vi "IVTcpLV2.vi"(4 "数值类型":enum16{"长整型", "双精度"}(ring), 6 "TCP连接参数":cluster{"IP地址":string, "端口":u16}={"IP地址"="10.232.43.160", "端口"=502}, 7 "TCP操作模式":enum16{"打开TCP", "读MW区", "写MW区", "关闭TCP"}(ring), 8 "错误输入":errorcluster, 9 "值":dbl format="%.3g", 10 "值":i32=10, 11 "寄存器MD地址":i32=10) -> (0 "错误输出":errorcluster, 1 "数值":sgl, 2 "数值":u32, 3 "=1？":bool)   [LabVIEW 2016]
panel:
  out "读写OK":bool
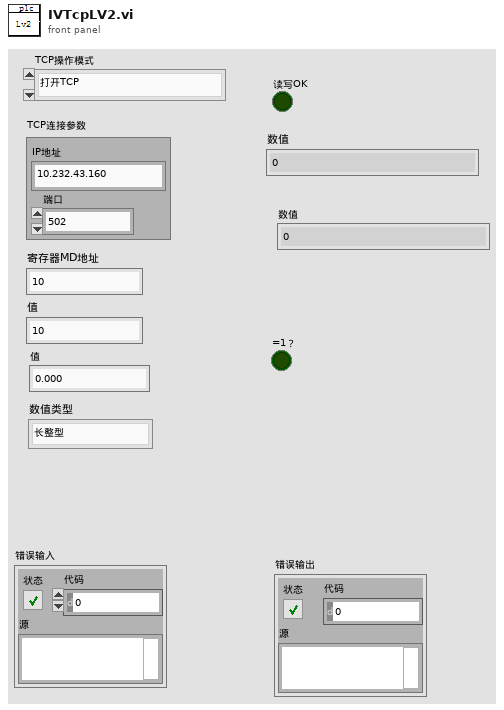
[diagram p1: front panel]
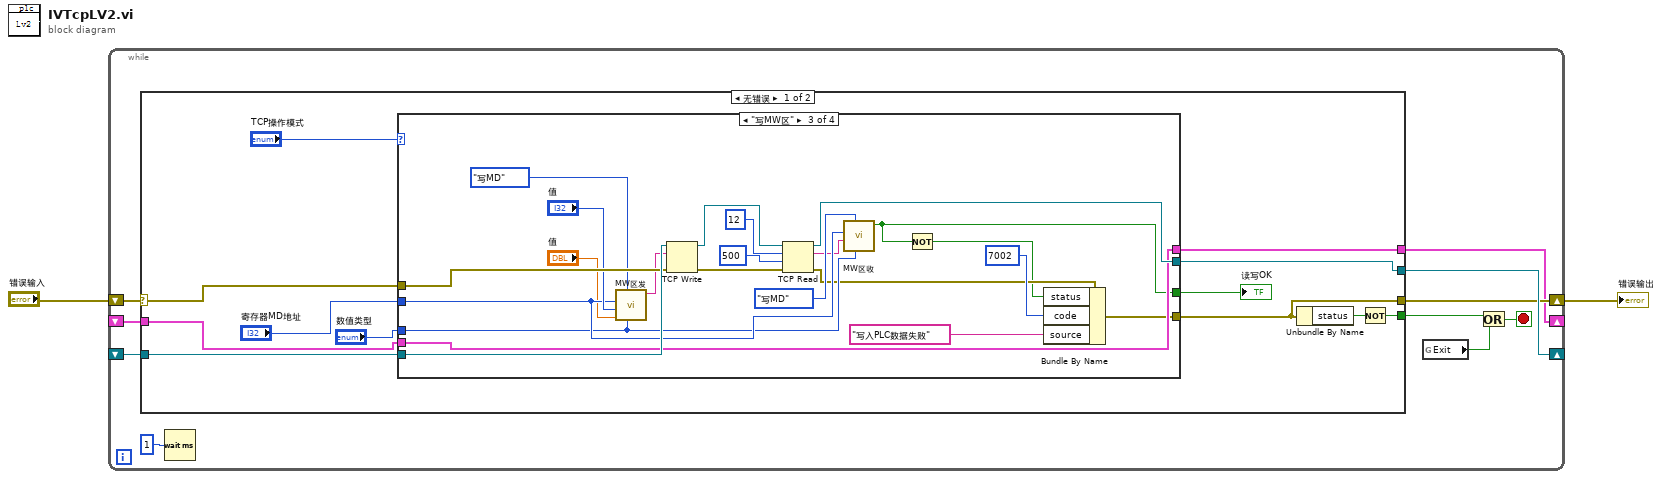
[diagram p0: block diagram]
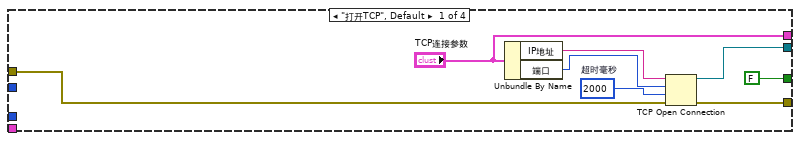
[diagram p2: hidden frame]
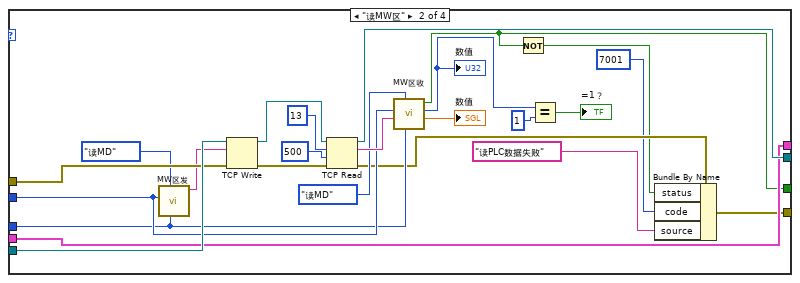
[diagram p3: hidden frame]
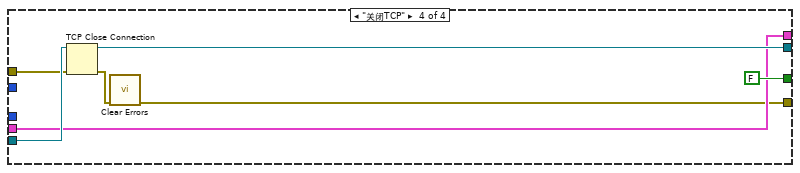
[diagram p4: hidden frame]
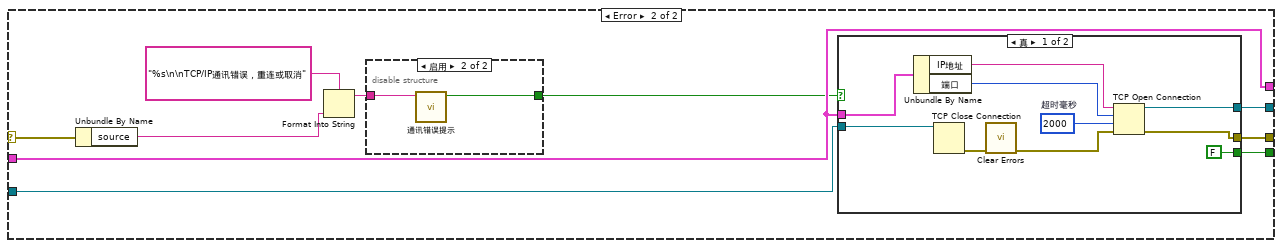
[diagram p5: hidden frame]
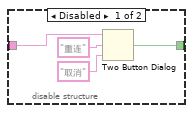
[diagram p6: hidden frame]
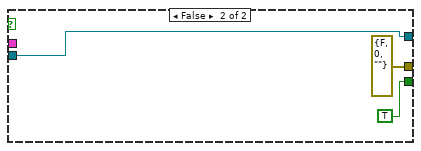
[diagram p7: hidden frame]
diagram:
  n1 = while {
    shift-right: [w6] -> w1
    shift-left: "错误输入" -> [w11]
    shift-right: [w10] -> _
    shift-left: _ -> [w12]
    shift-right: [w5] -> _
    shift-left: _ -> [w4]
    stop <- w8 stop-if-true
    n2 = case shown="无错误" w11 {
      selector: w11 -> [w18 w89]
      tunnel: w12 -> [w21 w94]
      tunnel: [w22 w95] -> w10
      tunnel: [w20 w93] -> w7
      tunnel: [w17 w92] -> w6
      tunnel: [w16 w91] -> w5
      tunnel: w4 -> [w15 w91]
      frame No Error {
        n3 = case shown="\"写MW区\"" "TCP操作模式" {
          tunnel: [FALSE ("读取OK") w36 w59 FALSE ("读取OK")] -> w24
          tunnel: [w31 w53 w74 w84] -> w22
          tunnel: w21 -> [_ w52 w75 w85]
          tunnel: [w30 w37 w57 w79] -> w17
          tunnel: w18 -> [w28 w51 w73 w81]
          tunnel: ["TCP连接参数" w50 w72 w82] -> w16
          tunnel: w15 -> [_ w50 w72 w82]
          tunnel: "寄存器MD地址" -> [_ w46 w67 _]
          tunnel: "数值类型" -> [_ w43 w63 _]
          frame "打开TCP", Default {
            w32 = 2000  # 超时毫秒
            n4 = Unbundle By Name("TCP连接参数") -> ("IP地址"=w27:string, "端口"=w26:u16)
            n5 = TCP Open Connection(address=w27, remote port or service name=w26, timeout ms (60000)=w32, error in (no error)=w28) -> (connection ID=w31:refnum<k5>, error out=w30:errorcluster)  [unwired: 1 in]
          }
          frame "读MW区" {
            n6 = call "MW区发.vi"("数值类型"=w43, "MD模式"=enum16{"读MD", "写MD"}."读MD", "寄存器MD地址"=w46) -> ("String"=w45:string)  [unwired: 8 in]
            n7 = TCP Write(connection ID=w52, data in=w45, error in (no error)=w51) -> (connection ID out=w56:refnum<k5>, error out=w55:errorcluster)  [unwired: 1 in, 1 out]
            n8 = TCP Read(connection ID=w56, bytes to read=13 ("读取的字节"), error in (no error)=w55, 9:500 ("超时毫秒(25000)")) -> (connection ID out=w53:refnum<k5>, data out=w48:string, error out=w38:errorcluster)  [unwired: 1 in]
            n9 = call "MW区收.vi"("数值类型"=w43, "MD模式"=enum16{"读MD", "写MD"}."读MD", "16#字符串"=w48, "寄存器MD地址"=w46) -> (1:"数值"=→"数值":sgl, 2:"数值"=w39:u32, "读写OK"=w36:bool)  [unwired: 5 in]
            "数值" <- w39
            n10 = Not(x=w36) -> (.not. x?=w35:bool)
            n11 = Equal?(x=w39, y=u32 1) -> (x = y?=→"=1？":bool)
            n12 = Bundle By Name(cluster=w38, "status"=w35, "code"=7001, "source"="读PLC数据失败") -> (w37:errorcluster)
          }
          frame "写MW区" {
            n13 = call "MW区发.vi"("数值类型"=w63, "MD模式"=enum16{"读MD", "写MD"}."写MD", 8:"值"="值", 9:"值"="值", "寄存器MD地址"=w67) -> ("String"=w69:string)  [unwired: 6 in]
            n14 = TCP Write(connection ID=w75, data in=w69, error in (no error)=w73) -> (connection ID out=w78:refnum<k5>, error out=w76:errorcluster)  [unwired: 1 in, 1 out]
            n15 = TCP Read(connection ID=w78, bytes to read=12 ("读取的字节"), error in (no error)=w76, 9:500 ("超时毫秒(25000)")) -> (connection ID out=w74:refnum<k5>, data out=w66:string, error out=w60:errorcluster)  [unwired: 1 in]
            n16 = call "MW区收.vi"("数值类型"=w63, "MD模式"=enum16{"读MD", "写MD"}."写MD", "16#字符串"=w66, "寄存器MD地址"=w67) -> ("读写OK"=w59:bool)  [unwired: 5 in, 2 out]
            n17 = Not(x=w59) -> (.not. x?=w58:bool)
            n18 = Bundle By Name(cluster=w60, "status"=w58, "code"=7002, "source"="写入PLC数据失败") -> (w57:errorcluster)
          }
          frame "关闭TCP" {
            n19 = TCP Close Connection(connection ID=w85, error in (no error)=w81) -> (connection ID out=w84:refnum<k5>, error out=w80:errorcluster)  [unwired: 1 in]
            n20 = call <vilib>:"Clear Errors.vi"("error in (no error)"=w80) -> ("error out"=w79:errorcluster)  [unwired: 5 in, 1 out]
          }
        }
        "读写OK" <- w24
        n21 = Unbundle By Name(w17) -> ("status"=w19:bool)
        n22 = Not(x=w19) -> (.not. x?=w20:bool)
      }
      frame Error {
        n23 = Unbundle By Name(w89) -> ("source"=w88:string)
        n24 = Format Into String(format string="%s\n\nTCP/IP通讯错误，重连或取消" ("消息"), w88) -> (resulting string=w86:string)  [unwired: 2 in, 1 out]
        n25 = disable-structure shown="启用" {
          disable-tunnel: [w97 w101] -> w90
          disable-tunnel: w86 -> [w96 w100]
          frame Disabled {
            n26 = Two Button Dialog(message=w96, 1:"取消" ("F按钮名称（“取消”）"), 2:"重连" ("T按钮名称（“确定”）")) -> (T button?=w97:bool)
          }
          frame Enabled {
            n27 = call "通讯错误提示.vi"("错误信息"=w100) -> ("重连？"=w101:bool)  [unwired: 10 in]
          }
        }
        n28 = case shown="真" w90 {
          tunnel: [FALSE ("status") TRUE ("status")] -> w93
          tunnel: [w107 errorcluster {"status"=FALSE, "code"=0, "source"=""} ("error out")] -> w92
          tunnel: [w106 w112] -> w95
          tunnel: w94 -> [w105 w112]
          tunnel: w91 -> [w104 _]
          frame True {
            w109 = 2000  # 超时毫秒
            n29 = Unbundle By Name(w104) -> ("IP地址"=w103:string, "端口"=w102:u16)
            n30 = TCP Close Connection(connection ID=w105) -> (error out=w110:errorcluster)  [unwired: 2 in, 1 out]
            n31 = call <vilib>:"Clear Errors.vi"("error in (no error)"=w110) -> ("error out"=w111:errorcluster)  [unwired: 5 in, 1 out]
            n32 = TCP Open Connection(address=w103, remote port or service name=w102, timeout ms (60000)=w109, error in (no error)=w111) -> (connection ID=w106:refnum<k5>, error out=w107:errorcluster)  [unwired: 1 in]
          }
          frame False {
          }
        }
      }
    }
    n33 = Wait (ms)(milliseconds to wait=u32 1 ("等待时间（毫秒）")) -> ()  [unwired: 1 out]
    n34 = global read "全局.vi" "Exit"() -> (w3:bool)
    n35 = Or(x=w7, y=w3) -> (x .or. y?=w8:bool)
  }
  "错误输出" <- w1
